vi "XIPIN_3GPP_LTE_MIMO_Decoder_3_0.vi"   [LabVIEW 2017]
doc: "The 3GPP LTE MIMO Decoder performs MIMO decoding using the MMSE algorithm. The core is fully synchronous, using a single clock, and integrates seamlessly with the Xilinx design flow.\n------------------------------------\n<b>Need License</b> : Yes"
uses:
  <vilib>/rvi/XilinxIP/XIPIN_XNode/niFpgaXIPIN.xnode
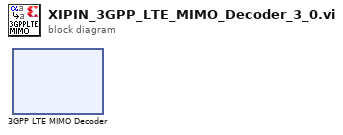
[diagram p0: block diagram]
diagram:
  n1 = xnode ("3GPP LTE MIMO Decoder")() -> ()
